vi "test_scd_OpenAndClose.vi"(8 "error in":errorcluster, 11 "SCD in":refnum<class "SCD.lvclass">) -> (0 "error out":errorcluster, 3 "SCD out":refnum<class "SCD.lvclass">)   [LabVIEW 2020, in "horiba.test.lvlib"]
uses:
  horiba.test.lvlib
  Classes/SCD/SCD.lvclass
  C:/Projects/Horiba/horiba-labview-sdk/Source/Classes/GenericDevice/GenericDevice.lvclass
  <vilib>/addons/_JKI Toolkits/Caraya/classes/Assert/Assert False.vi
  <vilib>/addons/_JKI Toolkits/Caraya/classes/Assert/Assert True.vi
  <vilib>/addons/_JKI Toolkits/Caraya/classes/Test/Test.lvclass
  <vilib>/addons/_JKI Toolkits/Caraya/classes/Assert/Assert.lvclass
  <userlib>/_OpenG.lib/lvdata/lvdata.llb/openg_variant.lvlib
panel:
  # "Connector Pane"
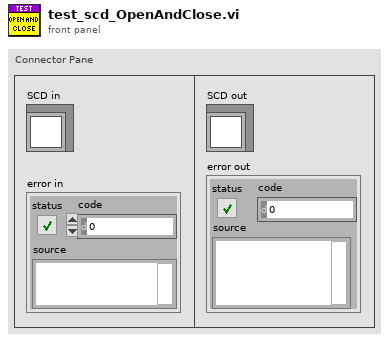
[diagram p1: front panel]
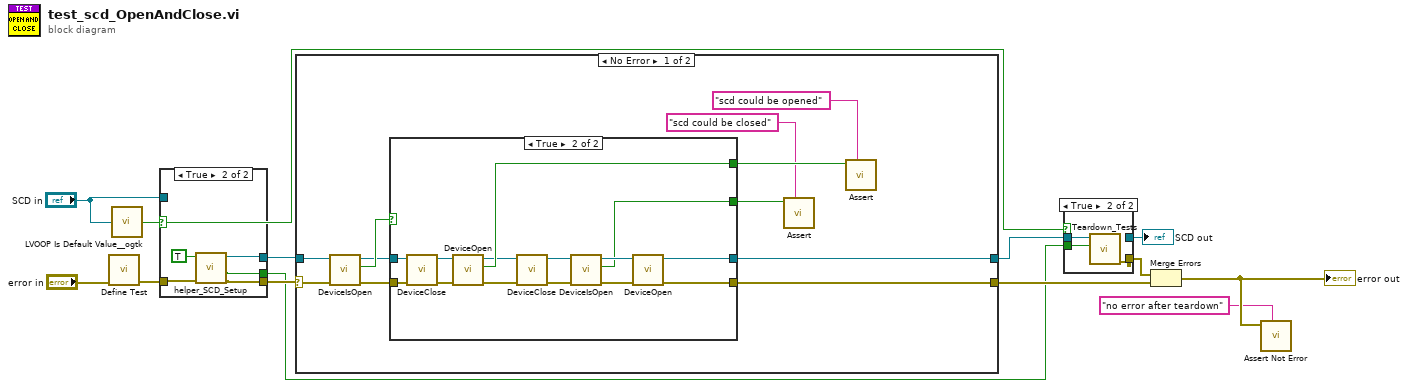
[diagram p0: block diagram]
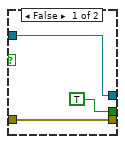
[diagram p3: hidden frame]
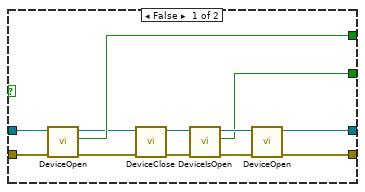
[diagram p4: hidden frame]
diagram:
  n1 = call <vilib>:"Define Test.vi"("error in (no error)"="error in") -> ("error out"=w9:errorcluster)  [unwired: 9 in, 1 out]
  n2 = call <userlib>:"LVOOP Is Default Value__ogtk.vi"("Object"="SCD in") -> ("Is Default Value?"=w3:bool)
  n3 = case shown="True" w3 {
    tunnel: w9 -> [w16 w19]
    tunnel: [w16 w21] -> w8
    tunnel: [w14 w18] -> w7
    tunnel: [TRUE ("Module Was Already Running?") w20] -> w4
    tunnel: "SCD in" -> [w14 _]
    frame False {
    }
    frame True {
      n4 = call "helper_SCD_Setup.vi"("error in"=w19, "show ICL for debugging"=TRUE) -> ("error out"=w21:errorcluster, "Module Was Already Running?"=w20:bool, "SCD out"=w18:refnum<class "SCD.lvclass">)  [unwired: 6 in, 1 out]
    }
  }
  n5 = case shown="No Error" w8 {
    selector: w8 -> [w31 w60]
    tunnel: [w22 w59] -> w12
    tunnel: w7 -> [w32 w59]
    tunnel: [w23 w60] -> w11
    frame No Error {
      n6 = call-dynamic "DeviceIsOpen.vi"("error in (no error)"=w31, "SCD in"=w32) -> ("error out"=w28:errorcluster, "device is open?"=w30:bool, "SCD out"=w29:refnum<class "SCD.lvclass">)  [unwired: 6 in, 1 out]
      n7 = case shown="True" w30 {
        tunnel: w29 -> [w43 w48]
        tunnel: w28 -> [w44 w49]
        tunnel: [w42 w58] -> w27
        tunnel: [w33 w45] -> w24
        tunnel: [w35 w51] -> w23
        tunnel: [w34 w50] -> w22
        frame False {
          n8 = call-dynamic "DeviceOpen.vi"("error in (no error)"=w44, "SCD in"=w43) -> ("error out"=w41:errorcluster, "device is open?"=w42:bool, "SCD out"=w40:refnum<class "SCD.lvclass">)  [unwired: 6 in, 1 out]
          n9 = call-dynamic "DeviceClose.vi"("error in (no error)"=w41, "SCD in"=w40) -> ("error out"=w39:errorcluster, "SCD out"=w38:refnum<class "SCD.lvclass">)  [unwired: 5 in, 3 out]
          n10 = call-dynamic "DeviceIsOpen.vi"("error in (no error)"=w39, "SCD in"=w38) -> ("error out"=w36:errorcluster, "device is open?"=w33:bool, "SCD out"=w37:refnum<class "SCD.lvclass">)  [unwired: 6 in, 1 out]
          n11 = call-dynamic "DeviceOpen.vi"("error in (no error)"=w36, "SCD in"=w37) -> ("error out"=w35:errorcluster, "SCD out"=w34:refnum<class "SCD.lvclass">)  [unwired: 6 in, 2 out]
        }
        frame True {
          n12 = call-dynamic "DeviceClose.vi"("error in (no error)"=w49, "SCD in"=w48) -> ("error out"=w46:errorcluster, "SCD out"=w47:refnum<class "SCD.lvclass">)  [unwired: 5 in, 3 out]
          n13 = call-dynamic "DeviceOpen.vi"("error in (no error)"=w46, "SCD in"=w47) -> ("error out"=w57:errorcluster, "device is open?"=w58:bool, "SCD out"=w56:refnum<class "SCD.lvclass">)  [unwired: 6 in, 1 out]
          n14 = call-dynamic "DeviceClose.vi"("error in (no error)"=w57, "SCD in"=w56) -> ("error out"=w55:errorcluster, "SCD out"=w54:refnum<class "SCD.lvclass">)  [unwired: 5 in, 3 out]
          n15 = call-dynamic "DeviceIsOpen.vi"("error in (no error)"=w55, "SCD in"=w54) -> ("error out"=w52:errorcluster, "device is open?"=w45:bool, "SCD out"=w53:refnum<class "SCD.lvclass">)  [unwired: 6 in, 1 out]
          n16 = call-dynamic "DeviceOpen.vi"("error in (no error)"=w52, "SCD in"=w53) -> ("error out"=w51:errorcluster, "SCD out"=w50:refnum<class "SCD.lvclass">)  [unwired: 6 in, 2 out]
        }
      }
      n17 = call-poly <vilib>:"Assert.vi"("Label"="scd could be closed", "False?"=w24) -> ()  [unwired: 8 in, 2 out]
      n18 = call-poly <vilib>:"Assert.vi"("Label"="scd could be opened", "True?"=w27) -> ()  [unwired: 8 in, 2 out]
    }
    frame Error {
    }
  }
  n19 = case shown="True" w3 {
    tunnel: w12 -> [w61 w64]
    tunnel: [_ w63] -> w6
    tunnel: w4 -> [_ w62]
    tunnel: [w61 _] -> w1
    frame False {
    }
    frame True {
      n20 = call "Teardown_Tests.vi"("Module Was Already Running?"=w62, "horiba.lvlib:GenericDevice"=w64) -> ("error out"=w63:errorcluster)  [unwired: 8 in, 1 out]
    }
  }
  "SCD out" <- w1
  n21 = Merge Errors(w6, w11) -> (w10:errorcluster)
  "error out" <- w10
  n22 = call <vilib>:"Assert Not Error.vi"("Label"="no error after teardown", "Not Error?"=w10) -> ()  [unwired: 8 in, 2 out]
